vi "Configure Connection UI.vi"(8 "error in (no error)":errorcluster) -> (0 "error out":errorcluster, 2 "Cancelled":bool, 3 "Configured Connection":refnum<class "Connection.lvclass">)   [LabVIEW 2020, in "LV-Term.lvlib" / "LV-Term App.lvclass"]
uses:
  LV-Term App.lvclass
  <vilib>/IlluminatedG/lv-stream/Connection/Connection.lvclass
  UI State.ctl
  ConfigPanel/ConfigPanel.lvclass
  C:/Program Files (x86)/National Instruments/LabVIEW 2020/vi.lib/IlluminatedG/IG OOPanel/OOPanel/Panel/Panel.lvclass
  <vilib>/IlluminatedG/lv-stream/Endpoint/Endpoint.lvclass
  <vilib>/IlluminatedG/IG OOPanel/OOPanel/Manager/Manager.lvclass
  <vilib>/Comparison/Equal/Equal Functor/Equal Functor.lvclass
  LV-Term App.lvclass/LV-Term App.ctl
panel:
  in  "Cancel Button":bool
  in  "OK Button":bool
  in  "Type":string(combo)
  # "Select a connection type to configure."
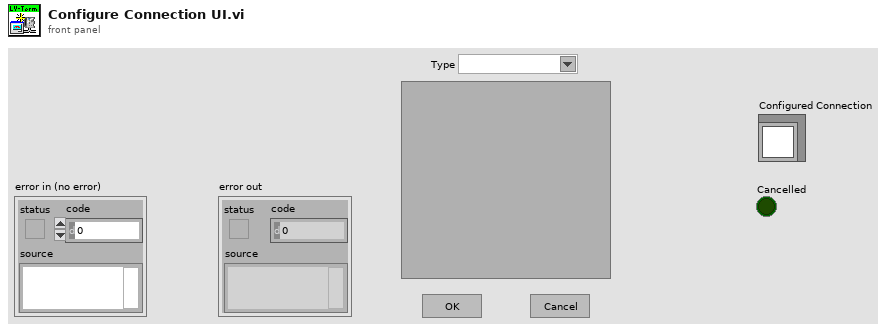
[diagram p1: front panel]
types:
  T1 = typedef "LV-Term.lvlib/LV-Term App.lvclass/UI State.ctl" = enum16{"Init", "Run", "Close"}
  T2 = enum8{"Enabled", "Disabled", "Disabled and Grayed Out"}
  T3 = typedef "LV-Term.lvlib/LV-Term App.lvclass/Available Type.ctl" = cluster{"Name":string, "Type":refnum<class "Endpoint.lvclass">, "Config":refnum<class "ConfigPanel.lvclass">}
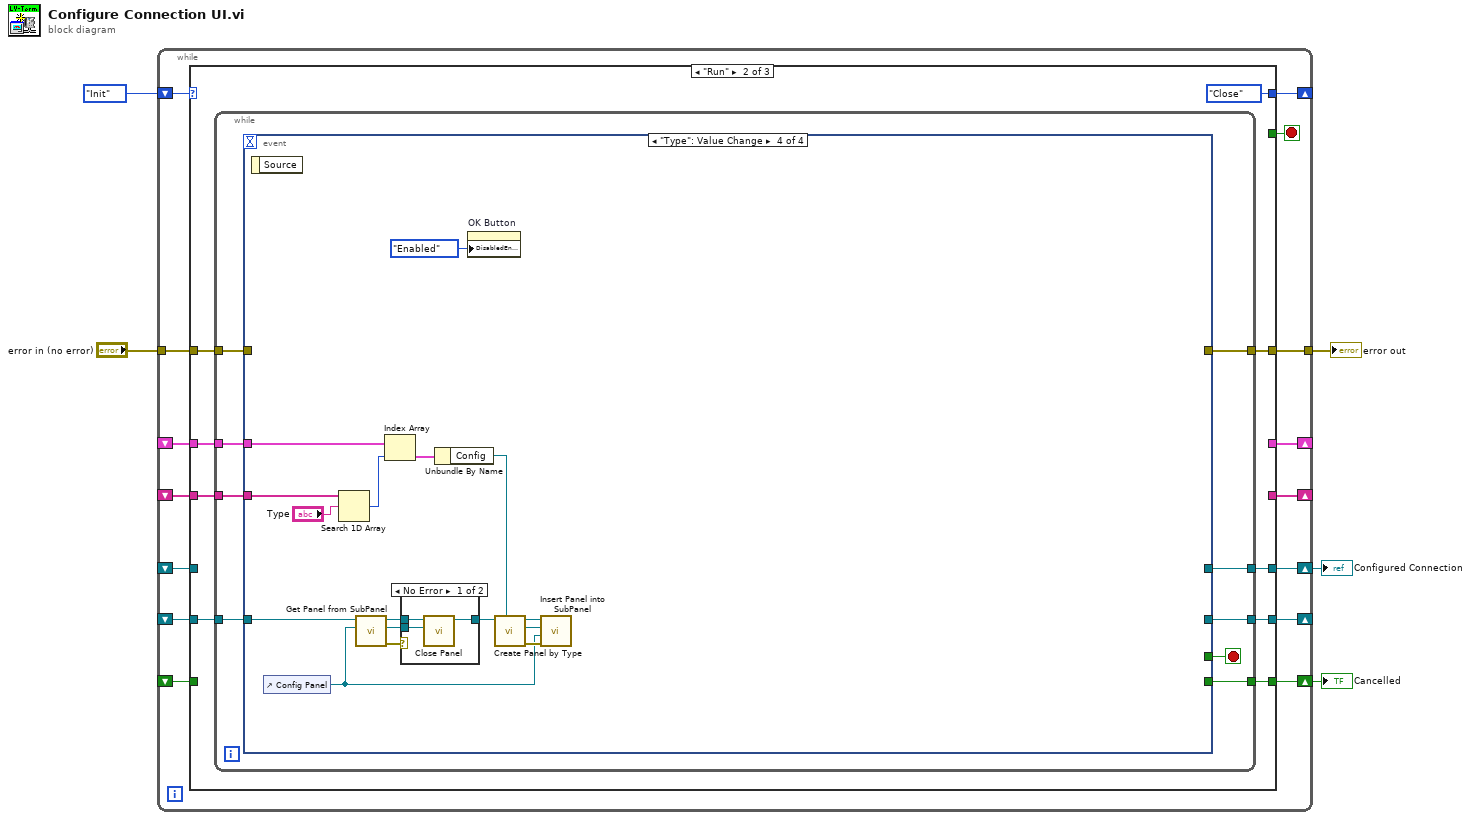
[diagram p0: block diagram]
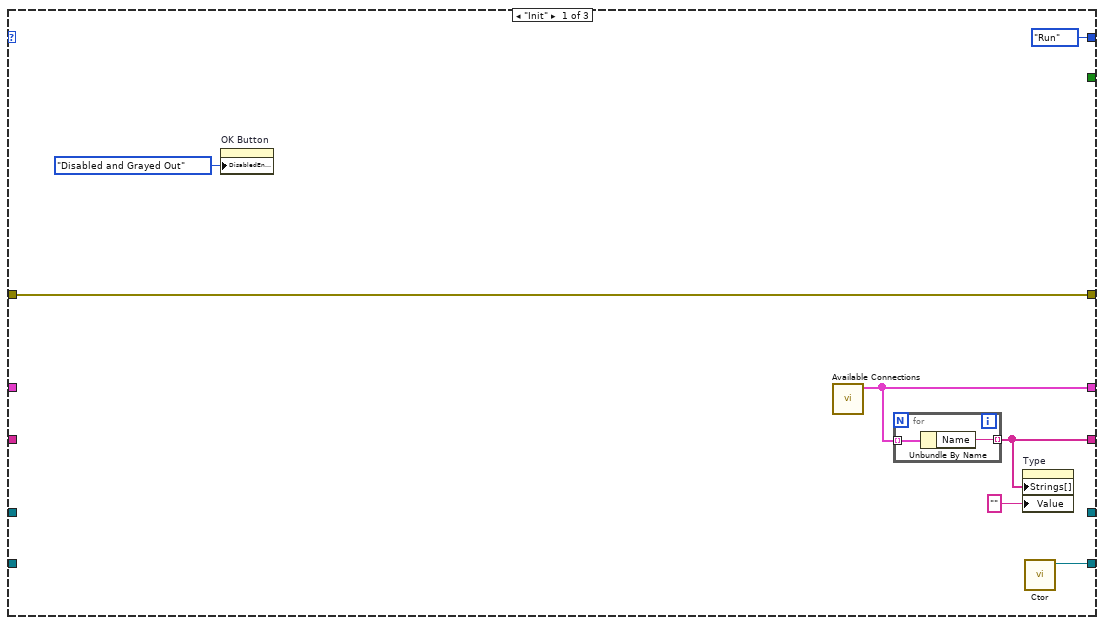
[diagram p2: hidden frame]
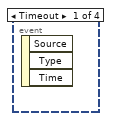
[diagram p3: hidden frame]
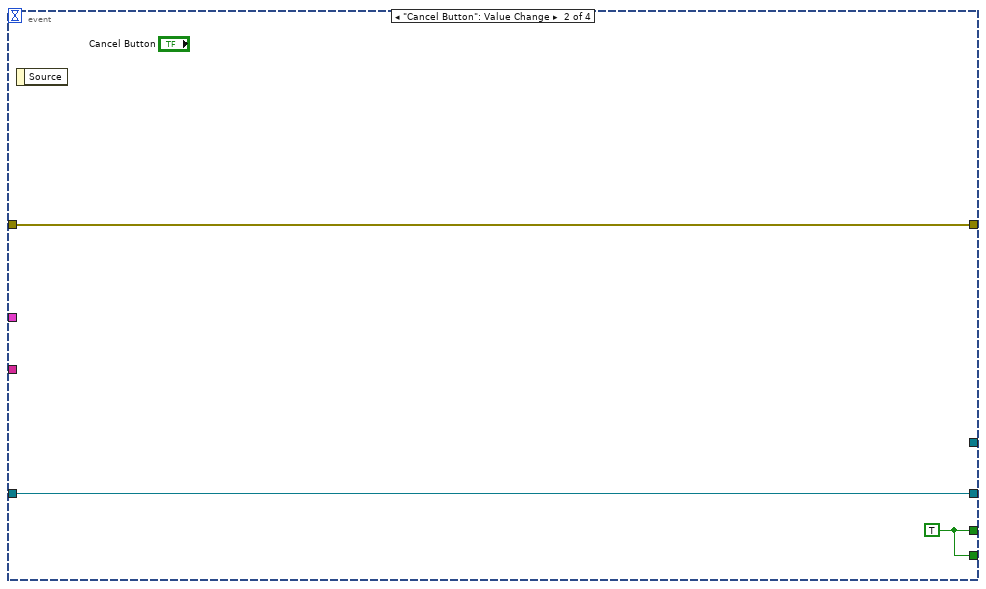
[diagram p4: hidden frame]
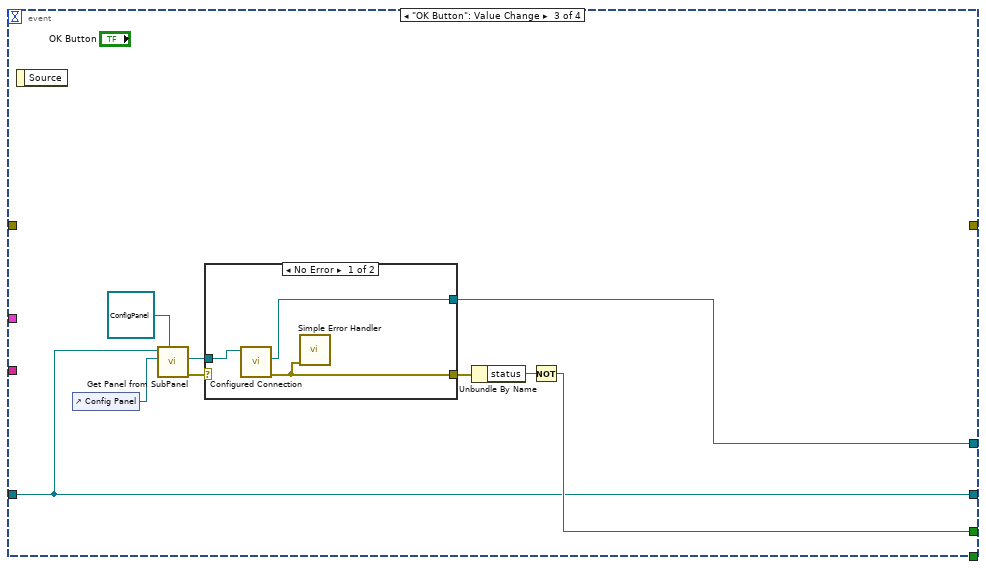
[diagram p5: hidden frame]
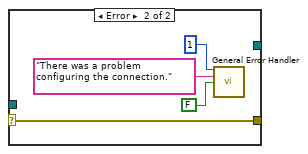
[diagram p6: hidden frame]
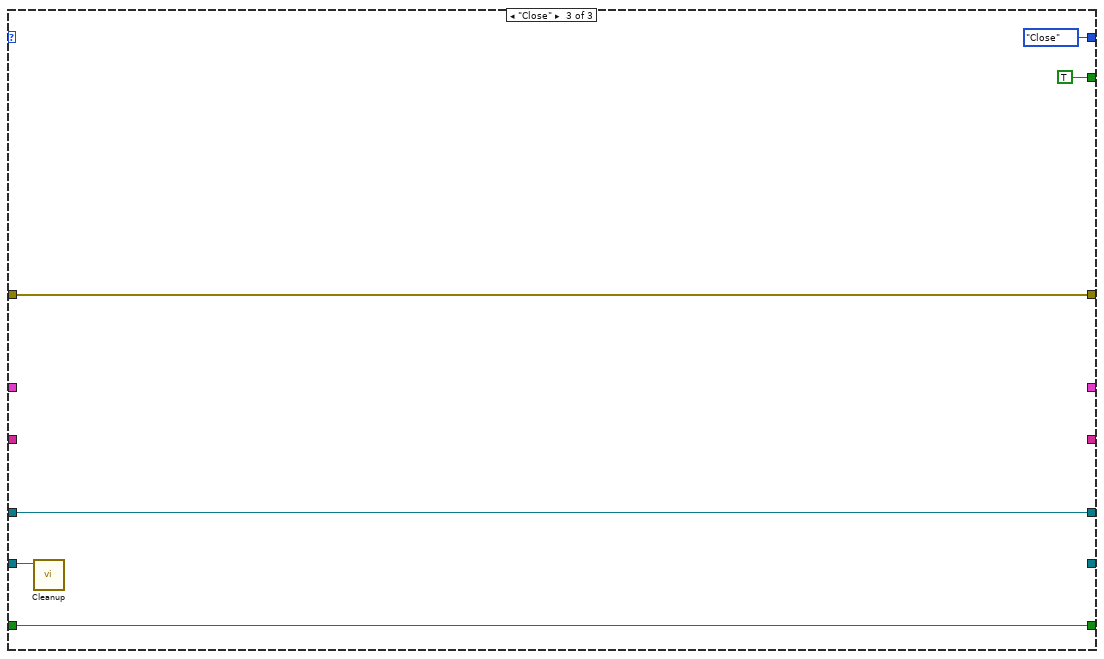
[diagram p8: hidden frame]
diagram:
  n1 = while {
    shift-right: [w19] -> _
    shift-left: UI_State."Init" ("UI State") -> [w20]
    tunnel: "error in (no error)" -> [w18]
    shift-right: [w17] -> _
    shift-left: _ -> [w16]
    tunnel: [w14] -> w3
    shift-right: [w13] -> _
    shift-left: _ -> [w12]
    shift-right: [w11] -> _
    shift-left: _ -> [w10]
    shift-right: [w9] -> w2
    shift-left: _ -> [w8]
    shift-right: [w7] -> w1
    shift-left: _ -> [w6]
    stop <- w15 stop-if-true
    n2 = case shown="\"Run\"" w20 {
      tunnel: [UI_State."Run" ("UI State") UI_State."Close" ("UI State") UI_State."Close" ("UI State")] -> w19
      tunnel: w18 -> [w24 w36 w90]
      tunnel: [w26 _ _] -> w17
      tunnel: w16 -> [_ w37 _]
      tunnel: [_ _ TRUE] -> w15
      tunnel: [w24 w32 w90] -> w14
      tunnel: [w23 _ _] -> w13
      tunnel: w12 -> [_ w35 _]
      tunnel: [w22 w33 _] -> w11
      tunnel: w10 -> [_ w34 w88]
      tunnel: [_ w31 w89] -> w9
      tunnel: w8 -> [_ _ w89]
      tunnel: [_ w30 w87] -> w7
      tunnel: w6 -> [_ _ w87]
      frame "Init" {
        n3 = property on="OK Button" class="Bool"("DisabledEnum"=T2."Disabled and Grayed Out" ("Disabled")) -> ()  [unwired: 2 in, 2 out]
        n4 = call "Available Connections.vi"() -> ("Available Types"=w26:T3[])  [unwired: 11 in]
        n5 = for {
          tunnel: w26 -> [w29] mode=indexing
          tunnel: [w28] -> w23 mode=indexing
          n6 = Unbundle By Name(w29) -> ("Name"=w28:string)
        }
        n7 = property on="Type" class="CmbBox"("Strings[]"=w23, "Value"="" ("Type")) -> ()  [unwired: 2 in, 2 out]
        n8 = call <vilib>:"Ctor.vi"() -> ("Manager out"=w22:refnum<class "Manager.lvclass">)  [unwired: 10 in, 1 out]
      }
      frame "Run" {
        n9 = while {
          tunnel: w37 -> [w46]
          tunnel: w36 -> [w47]
          tunnel: w35 -> [w45]
          tunnel: w34 -> [w44]
          tunnel: [w42] -> w33
          tunnel: [w41] -> w32
          tunnel: [w40] -> w31
          tunnel: [w39] -> w30
          stop <- w43 stop-if-true
          n10 = event shown="[3] \"Type\": Value Change" {
            selector: _ -> [_ _ _ _]
            dyn-events: _ -> [_ _ _ _]
            timeout: _ -> [_ _ _ _]
            tunnel: w47 -> [_ w49 _ _]
            tunnel: w46 -> [_ _ _ w82]
            tunnel: w45 -> [_ _ _ w69]
            tunnel: w44 -> [_ w50 w51 w80]
            tunnel: [_ w48 w52 _] -> w43
            tunnel: [_ w50 w51 _] -> w42
            tunnel: [_ w49 _ _] -> w41
            tunnel: [_ _ w55 _] -> w40
            tunnel: [_ w48 _ _] -> w39
            event Timeout {
              n11 = event-data() -> ()  [unwired: 1 in, 3 out]
            }
            event "Cancel Button": Value Change {
              w48 = TRUE
              n12 = event-data() -> ()  [unwired: 1 in, 1 out]
            }
            event "OK Button": Value Change {
              n13 = event-data() -> ()  [unwired: 1 in, 1 out]
              n14 = control-ref of="Config Panel"() -> (w59:refnum<vi>)
              n15 = call <vilib>:"Get Panel from SubPanel.vi"("Panel Type (Panel)"=refnum<class "ConfigPanel.lvclass"> refnum ("LV-Term.lvlib:ConfigPanel.lvclass"), "SubPanel"=w59, "Manager in"=w51) -> ("error out"=w57:errorcluster, "Panel"=w56:refnum<class "ConfigPanel.lvclass">)  [unwired: 6 in, 1 out]
              n16 = case shown="No Error" w57 {
                selector: w57 -> [_ w63]
                tunnel: w56 -> [w62 _]
                tunnel: [w60 w63] -> w54
                tunnel: [w61 _] -> w55
                frame No Error {
                  n17 = call-dynamic "Configured Connection.vi"("ConfigPanel in"=w62) -> ("error out"=w60:errorcluster, "Configured Connection"=w61:refnum<class "Connection.lvclass">)  [unwired: 8 in, 1 out]
                  n18 = call <vilib>:"Simple Error Handler.vi"("error in (no error)"=w60) -> ()  [unwired: 4 in, 5 out]
                }
                frame Error {
                  n19 = call <vilib>:"General Error Handler.vi"("[error code] (0)"=1, "[error source] (\" \")"="There was a problem configuring the connection." ("[error source] (\" \")"), "search ni.com link visible?(T)"=FALSE) -> ()  [unwired: 8 in, 5 out]
                }
              }
              n20 = Unbundle By Name(w54) -> ("status"=w53:bool)
              n21 = Not(x=w53) -> (.not. x?=w52:bool)
            }
            event "Type": Value Change {
              n22 = event-data() -> ()  [unwired: 1 in, 1 out]
              n23 = control-ref of="Config Panel"() -> (w70:refnum<vi>)
              n24 = Search 1D Array(1D array=w69, element="Type") -> (index of element=w67:i32)  [unwired: 1 in]
              n25 = call <vilib>:"Get Panel from SubPanel.vi"("SubPanel"=w70, "Manager in"=w80) -> ("error out"=w79:errorcluster, "Panel"=w77:refnum<class "Panel.lvclass">, "Manager out"=w78:refnum<class "Manager.lvclass">)  [unwired: 7 in]
              n26 = Index Array(array=w82, index=w67) -> (element=w76:T3)
              n27 = case shown="No Error" w79 {
                tunnel: w78 -> [w85 w86]
                tunnel: w77 -> [w84 _]
                tunnel: [w83 w86] -> w75
                frame No Error {
                  n28 = call <vilib>:"Close Panel.vi"("Panel"=w84, "Manager in"=w85) -> ("Manager out"=w83:refnum<class "Manager.lvclass">)  [unwired: 8 in, 1 out]
                }
                frame Error {
                }
              }
              n29 = Unbundle By Name(w76) -> ("Config"=w74:refnum<class "ConfigPanel.lvclass">)
              n30 = property on="OK Button" class="Bool"("DisabledEnum"=T2."Enabled" ("Disabled")) -> ()  [unwired: 2 in, 2 out]
              n31 = call <vilib>:"Create Panel by Type.vi"("Panel Type"=w74, "Manager in"=w75) -> ("error out"=w71:errorcluster, "Panel"=w72:refnum<class "ConfigPanel.lvclass">, "Manager out"=w73:refnum<class "Manager.lvclass">)  [unwired: 7 in]
              n32 = call <vilib>:"Insert Panel into SubPanel.vi"("error in (no error)"=w71, "SubPanel"=w70, "Panel In"=w72, "Manager in"=w73) -> ()  [unwired: 5 in, 3 out]
            }
          }
        }
      }
      frame "Close" {
        n33 = call <vilib>:"Cleanup.vi"("Manager in"=w88) -> ()  [unwired: 8 in, 3 out]
      }
    }
  }
  "error out" <- w3
  "Configured Connection" <- w2
  "Cancelled" <- w1
